vi "Load Data V1.00.vi"(4 "Wavelength Unit Used in the Plot":i32(ring)=1 items=["Wavelength", "nm", "eV", "meV", "cm-1"]) -> (0 "Data Array output":dbl[][](array[numeric]) format="%.2f", 1 "X-Axis Array output":dbl[][](array[numeric]) format="%.2f")   [LabVIEW 2019]
uses:
  <vilib>/Utility/file.llb/Read From Spreadsheet File (DBL).vi
panel:
  out "File Contents":string
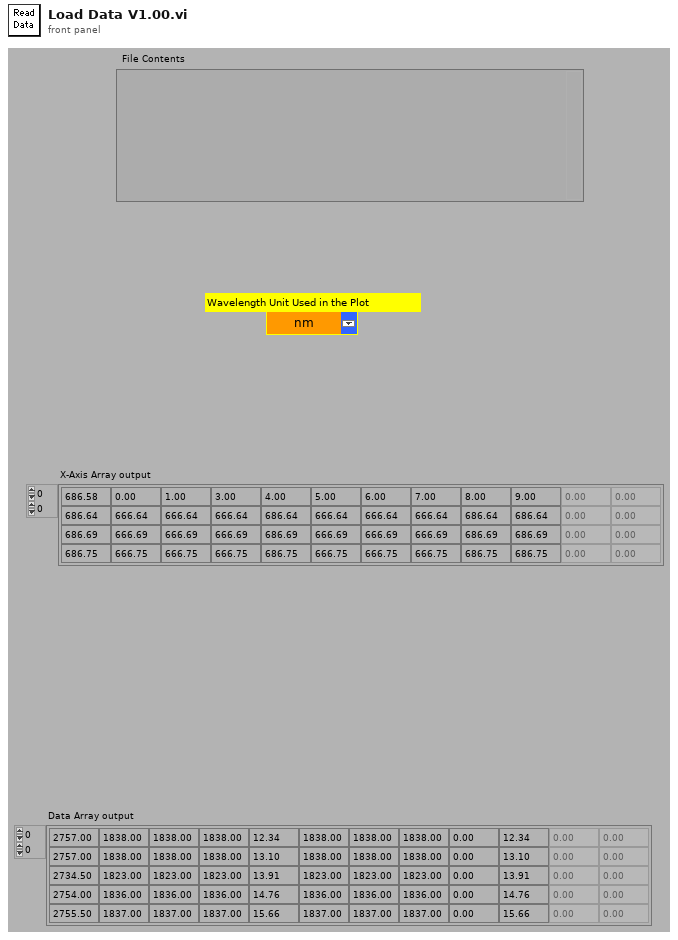
[diagram p1: front panel]
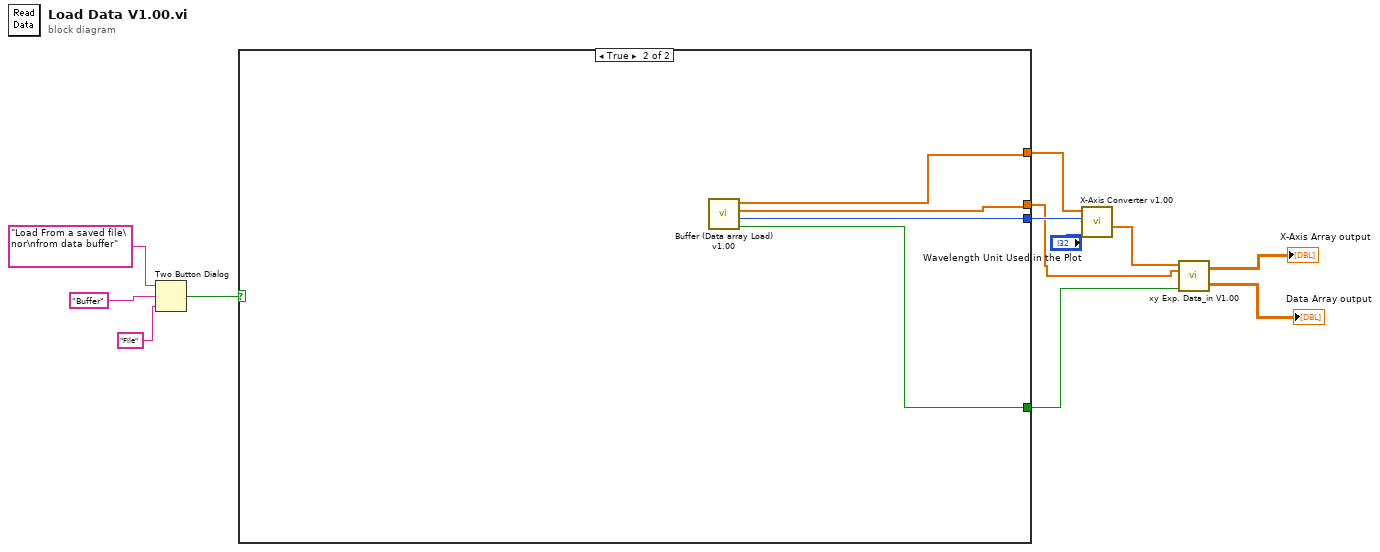
[diagram p0: block diagram]
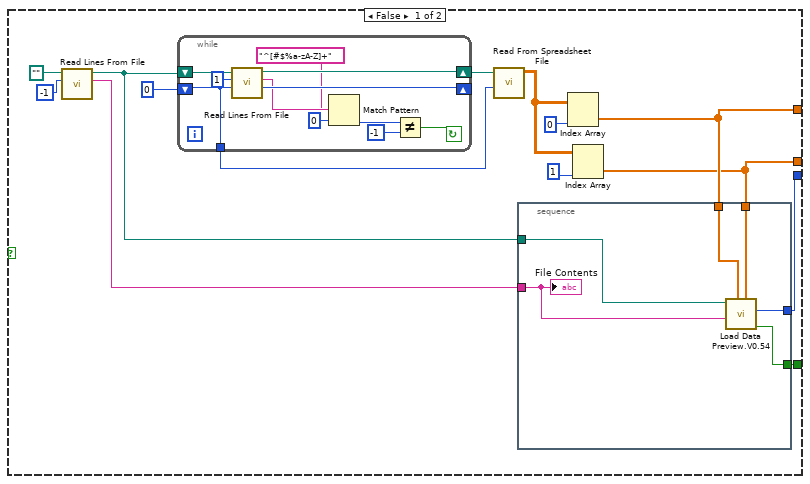
[diagram p2: hidden frame]
diagram:
  n1 = Two Button Dialog(message="Load From a saved file\nor\nfrom data buffer", 1:"File" ("F button name (\"Cancel\")"), 2:"Buffer" ("T button name (\"OK\")")) -> (T button?=w9:bool)
  n2 = case shown="True" w9 {
    tunnel: [w22 w44] -> w3
    tunnel: [w21 w45] -> w12
    tunnel: [w14 w47] -> w11
    tunnel: [w13 w46] -> w10
    frame False {
      n3 = call <vilib>:"Read Lines From File.vi"("file path (dialog if empty)"=path "", "number of lines (all:-1)"=-1) -> ("new file path (Not A Path if cancelled)"=w20:path, "line string"=w23:string)  [unwired: 4 in, 2 out]
      n4 = while {
        tunnel: [w27] -> w15
        shift-left: 0 ("mark after read (chars.)") -> [w27]
        shift-right: [w34] -> _
        shift-left: w20 -> [w37]
        shift-right: [w36] -> w16
        stop <- w30 continue-if-true
        n5 = call <vilib>:"Read Lines From File.vi"("file path (dialog if empty)"=w37, "number of lines (all:-1)"=1, "start of read offset (chars.:0)"=w27) -> ("new file path (Not A Path if cancelled)"=w36:path, "line string"=w33:string, "mark after read (chars.)"=w34:i32)  [unwired: 3 in, 1 out]
        n6 = Match Pattern(string=w33, regular expression="^[#$%a-zA-Z]+", offset (0)=0) -> (offset past match=w29:i32)  [unwired: 3 out]
        n7 = Not Equal?(x=w29, y=-1) -> (x != y?=w30:bool)
      }
      n8 = call-poly <vilib>:"Read From Spreadsheet File.vi"("start of read offset (chars.:0)"=w15, "file path (dialog if empty)"=w16) -> ("all rows"=w19:dbl[][])  [unwired: 5 in, 4 out]
      n9 = Index Array(array=w19, index (col)=0) -> (element=w14:dbl[])  [unwired: 1 in]
      n10 = Index Array(array=w19, index (col)=1) -> (element=w13:dbl[])  [unwired: 1 in]
      n11 = stacked-sequence {
        tunnel: w23 -> [w43]
        tunnel: [w42] -> w22
        tunnel: [w41] -> w21
        tunnel: w20 -> [w40]
        tunnel: w14 -> [w39]
        tunnel: w13 -> [w38]
        frame #0 {
          n12 = call "Load Data Preview.V0.54.vi"("Y-Array"=w38, "X-Array"=w39, "File Contents"=w43, "File Path"=w40) -> ("Continue?"=w42:bool, "WL unit copy"=w41:i32)  [unwired: 4 in]
          "File Contents" <- w43
        }
      }
    }
    frame True {
      n13 = call "Buffer (Data array Load) v1.00.vi"() -> ("X-Data out"=w47:dbl[], "Y-Data out"=w46:dbl[], "WL unit 2"=w45:i32, "Continue? 2"=w44:bool)  [unwired: 2 in]
    }
  }
  n14 = call "X-Axis Converter v1.00.vi"("X-Axis Unit"="Wavelength Unit Used in the Plot", "Old X-Axis Unit"=w12, "X-Axis input"=w11) -> ("X-Axis Output"=w4:dbl[])  [unwired: 2 in, 3 out]
  n15 = call "xy Exp. Data_in V1.00.vi"("X-axis row"=w4, "Data row"=w10, "Continue?"=w3) -> ("X-Axis Array"=→"X-Axis Array output":dbl[][], "Data Array"=→"Data Array output":dbl[][])  [unwired: 2 in]
